vi "Set Password.vi"(11 "Ini File":path=path "D:/LABVIEW/SEQUENSER_SNA/Ver_12/INI/SysConfig.ini") -> (2 "Password":string, 3 "Password Ok":bool)   [LabVIEW 2018]
uses:
  <vilib>/Utility/miscctls.llb/LVSelectionTypeDef.ctl
  <vilib>/Utility/config.llb/Read Key (U32).vi
  <vilib>/Utility/config.llb/Read Key (String).vi
  <vilib>/Utility/config.llb/NI_LVConfig.lvlib
panel:
  out "Exit":bool
  out "Value":string
  out "Length":u32
  in  "stop":bool
  out "Key Focus":bool
  in  "Password In":string="****"
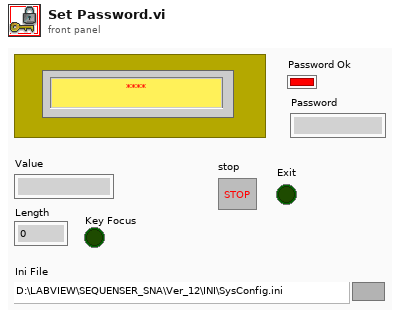
[diagram p1: front panel]
types:
  T1 = enum32{"Invalid", "Standard", "Closed", "Hidden", "Minimized", "Maximized"}
  T2 = enum32{"Invalid", "Default", "Floating", "Floating/Auto-Hide", "Modal"}
  T3 = typedef "LVSelectionTypeDef.ctl" = cluster{"Selection Start":u32, "Selection End":u32}
  T4 = typedef "NI_LVConfig.lvlib/Config Data RefNum.ctl" = refnum<k1>
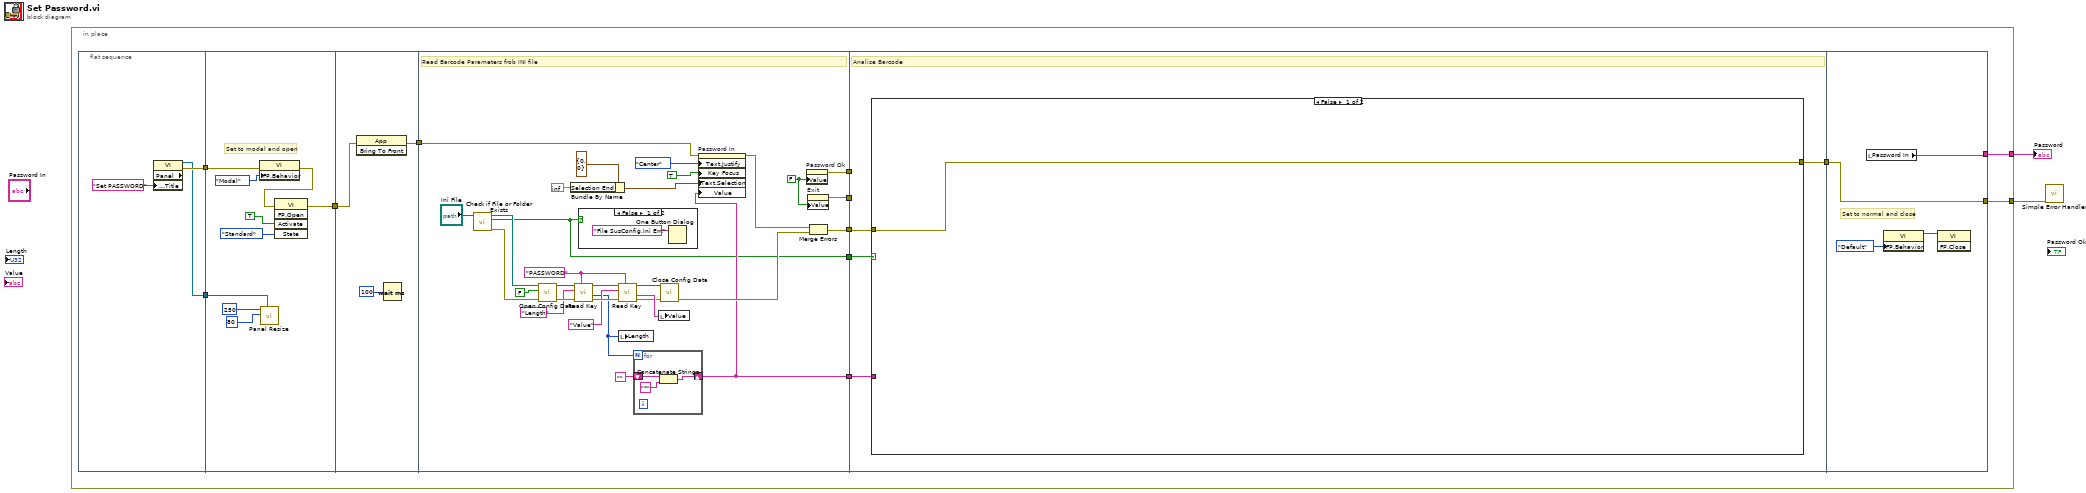
[diagram p0: block diagram]
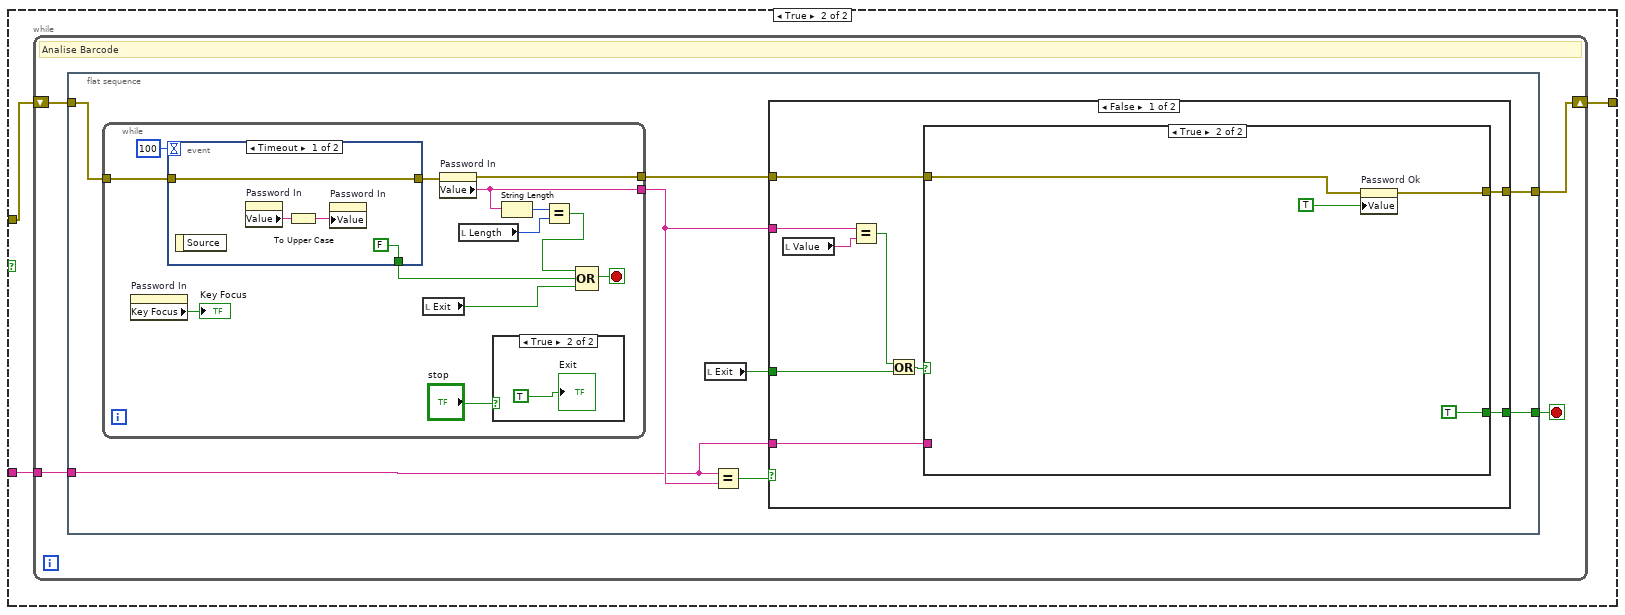
[diagram p3: hidden frame]
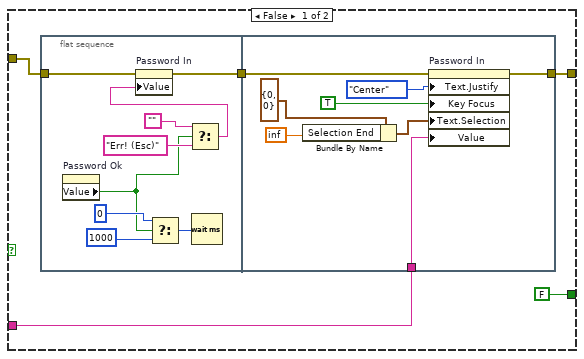
[diagram p4: hidden frame]
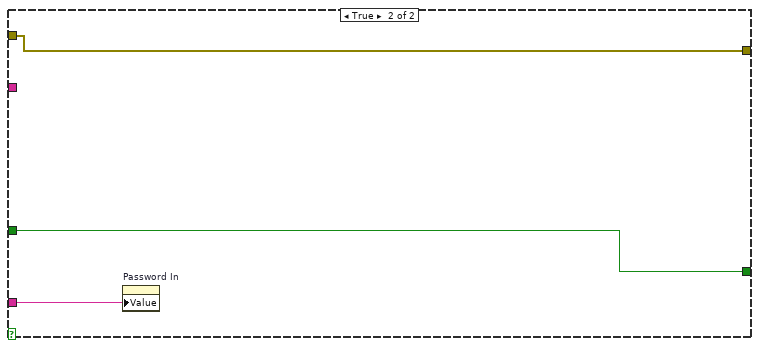
[diagram p5: hidden frame]
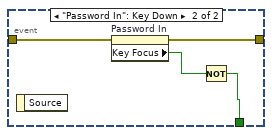
[diagram p7: hidden frame]
diagram:
  n1 = in-place {
    in-place-border: [w9] -> w2
    in-place-border: [w8] -> w1
    n2 = flat-sequence {
      tunnel: [w16] -> w14
      tunnel: [w15] -> w13
      tunnel: [w23] -> w12
      tunnel: w14 -> [w22]
      tunnel: w13 -> [w20]
      tunnel: [w29] -> w11
      tunnel: w12 -> [w27]
      tunnel: w11 -> [w45]
      tunnel: [w51] -> w10
      tunnel: [w44] -> w6
      tunnel: [w34] -> w5
      tunnel: [w32] -> w4
      tunnel: [w31] -> w3
      tunnel: w10 -> [w67]
      tunnel: [w66] -> w7
      tunnel: w6 -> [_]
      tunnel: w5 -> [w65]
      tunnel: w4 -> [_]
      tunnel: w3 -> [w64]
      tunnel: [w144] -> w9
      tunnel: [w146] -> w8
      tunnel: w7 -> [w144]
      frame #0 {
        n3 = property class="VI" props=["Panel", "Front Panel.Title"]("Front Panel.Title"="Set PASSWORD" ("Front Panel Window:Title")) -> (reference out=w15:refnum<vi>, error out=w16:errorcluster)  [unwired: 2 in, 1 out]
      }
      frame #1 {
        # "Set to modal and open"
        n4 = property class="VI"(error in=w22, "FP.Behavior"=T2."Modal" ("Front Panel Window:Behavior")) -> (error out=w26:errorcluster)  [unwired: 1 in, 1 out]
        n5 = call "Panel Resize.vi"("Width"=i16 250, "Height"=i16 80, "reference"=w20) -> ()  [unwired: 7 in, 1 out]
        n6 = invoke class="VI" method="FP.Open"(error in=w26, "Activate"=TRUE ("Activate?"), "State"=T1."Standard") -> (error out=w23:errorcluster)  [unwired: 2 in, 4 out]
      }
      frame #2 {
        n7 = invoke class="App" method="Bring To Front"(error in=w27) -> (error out=w29:errorcluster)  [unwired: 2 in, 2 out]
        n8 = Wait (ms)(milliseconds to wait=u32 100) -> ()  [unwired: 1 out]
      }
      frame #3 {
        w33 = FALSE ("Exit")
        w54 = "PASSWORD"
        # "Read Barcode Parameters frob INI file"
        n9 = call <vilib>:"Check if File or Folder Exists.vi"("path"="Ini File") -> ("error out"=w57:errorcluster, "file or folder exists?"=w31:bool, "dup path"=w58:path)  [unwired: 8 in]
        n10 = call <vilib>:"Open Config Data.vi"("error in (no error)"=w57, "create file if necessary (T)"=FALSE, "configuration file path"=w58) -> ("error out"=w52:errorcluster, "refnum"=w56:T4)  [unwired: 6 in, 1 out]
        n11 = Bundle By Name(cluster=T3 {"Selection Start"=0, "Selection End"=0} ("Text.Selection"), "Selection End"=inf) -> (w38:T3)
        n12 = call-poly <vilib>:"Read Key.vi"("section"=w54, "error in (no error)"=w52, "key"="Length", "refnum"=w56) -> ("error out"=w53:errorcluster, "value"=w36:u32, "refnum out"=w55:T4)  [unwired: 4 in, 1 out]
        n13 = case shown="False" w31 {
          frame False {
            n14 = One Button Dialog(message="File SusConfig.Ini Err!") -> ()  [unwired: 1 in, 1 out]
          }
          frame True {
          }
        }
        n15 = call-poly <vilib>:"Read Key.vi"("section"=w54, "error in (no error)"=w53, "key"="Value", "refnum"=w55) -> ("error out"=w42:errorcluster, "value"=w46:string, "refnum out"=w43:T4)  [unwired: 4 in, 1 out]
        n16 = local write "Length"(w36) -> ()
        n17 = for {
          N: w36 -> [_]
          shift-right: [w61] -> w34
          shift-left: "" -> [w62]
          n18 = Concatenate Strings(w62, "*") -> (w61:string)
        }
        n19 = local write "Value"(w46) -> ()
        n20 = call <vilib>:"Close Config Data.vi"("error in (no error)"=w42, "refnum"=w43) -> ("error out"=w49:errorcluster)  [unwired: 8 in, 1 out]
        n21 = property on="Password In" class="Str"(error in=w45, "Text.Justify"=enum16{"Left", "Center", "Right"}."Center" ("Text.Justification"), "Key Focus"=TRUE, "Text.Selection"=w38, "Value"=w34) -> (error out=w50:errorcluster)  [unwired: 1 in, 1 out]
        n22 = property on="Password Ok" class="Bool (strict)"("Value"=w33) -> (error out=w44:errorcluster)  [unwired: 2 in, 1 out]
        n23 = property on="Exit" class="Bool (strict)"("Value"=w33) -> (error out=w32:errorcluster)  [unwired: 2 in, 1 out]
        n24 = Merge Errors(w50, w49) -> (w51:errorcluster)
      }
      frame #4 {
        # "Analise Barcode"
        n25 = case shown="False" w64 {
          tunnel: w67 -> [w68 w71]
          tunnel: [w68 w70] -> w66
          tunnel: w65 -> [_ w69]
          frame False {
          }
          frame True {
            n26 = while {
              shift-right: [w73] -> w70
              shift-left: w71 -> [w75]
              tunnel: w69 -> [w72]
              stop <- w74 stop-if-true
              # "Analise Barcode"
              n27 = flat-sequence {
                tunnel: [w82] -> w74
                tunnel: [w81] -> w73
                tunnel: w75 -> [w83]
                tunnel: w72 -> [w77]
                frame #0 {
                  n28 = while {
                    tunnel: w83 -> [w132]
                    tunnel: [w129] -> w80
                    tunnel: [w128] -> w78
                    stop <- w123 stop-if-true
                    n29 = property on="Password In" class="Str"() -> ("Key Focus"=→"Key Focus":bool)  [unwired: 2 in, 2 out]
                    n30 = event shown="[0] Timeout" {
                      selector: _ -> [_ _]
                      dyn-events: _ -> [_ _]
                      timeout: 100 -> [_ _]
                      tunnel: [FALSE w142] -> w124
                      tunnel: w132 -> [w136 w141]
                      tunnel: [w136 w140] -> w130
                      event Timeout {
                        n31 = event-data() -> ()  [unwired: 1 in, 1 out]
                        n32 = property on="Password In" class="Str"() -> ("Value"=w139:string)  [unwired: 2 in, 2 out]
                        n33 = To Upper Case(1:w139) -> (0:w138:string)
                        n34 = property on="Password In" class="Str"("Value"=w138) -> ()  [unwired: 2 in, 2 out]
                      }
                      event "Password In": Key Down {
                        n35 = event-data() -> ()  [unwired: 1 in, 1 out]
                        n36 = property on="Password In" class="Str"(error in=w141) -> (error out=w140:errorcluster, "Key Focus"=w143:bool)  [unwired: 1 in, 1 out]
                        n37 = Not(x=w143) -> (.not. x?=w142:bool)
                      }
                    }
                    n38 = local read "Exit"() -> (w122:bool)
                    n39 = property on="Password In" class="Str"(error in=w130) -> (error out=w129:errorcluster, "Value"=w128:string)  [unwired: 1 in, 1 out]
                    n40 = local read "Length"() -> (w126:u32)
                    n41 = case shown="True" "stop" {
                      frame False {
                      }
                      frame True {
                        "Exit" <- TRUE ("Exit")
                      }
                    }
                    n42 = String Length(string=w128) -> (length=w127:i32)
                    n43 = Equal?(x=w127, y=w126) -> (x = y?=w125:bool)
                    n44 = Compound Arithmetic op=OR(w125, w124, w122) -> (w123:bool)
                  }
                  n45 = local read "Exit"() -> (w76:bool)
                  n46 = Equal?(x=w77, y=w78) -> (x = y?=w79:bool)
                  n47 = case shown="False" w79 {
                    tunnel: [w92 w119] -> w82
                    tunnel: [w91 w121] -> w81
                    tunnel: w80 -> [w89 w121]
                    tunnel: w78 -> [w88 _]
                    tunnel: w76 -> [w85 w119]
                    tunnel: w77 -> [w84 w120]
                    frame False {
                      n48 = local read "Value"() -> (w87:string)
                      n49 = Equal?(x=w88, y=w87) -> (x = y?=w86:bool)
                      n50 = Or(x=w86, y=w85) -> (x .or. y?=w90:bool)
                      n51 = case shown="True" w90 {
                        tunnel: [FALSE TRUE] -> w92
                        tunnel: [w96 w117] -> w91
                        tunnel: w89 -> [w94 w116]
                        tunnel: w84 -> [w93 _]
                        frame False {
                          n52 = flat-sequence {
                            tunnel: [w106] -> w95
                            tunnel: w94 -> [w105]
                            tunnel: [w112] -> w96
                            tunnel: w95 -> [w111]
                            tunnel: w93 -> [w107]
                            frame #0 {
                              n53 = property on="Password Ok" class="Bool (strict)"() -> ("Value"=w98:bool)  [unwired: 2 in, 2 out]
                              n54 = Select(t=u32 0 ("milliseconds to wait"), s=w98, f=u32 1000 ("milliseconds to wait")) -> (s? t:f=w101:u32)
                              n55 = Select(t="", s=w98, f="Err! (Esc)") -> (s? t:f=w104:string)
                              n56 = property on="Password In" class="Str"(error in=w105, "Value"=w104) -> (error out=w106:errorcluster)  [unwired: 1 in, 1 out]
                              n57 = Wait (ms)(milliseconds to wait=w101) -> ()  [unwired: 1 out]
                            }
                            frame #1 {
                              n58 = Bundle By Name(cluster=T3 {"Selection Start"=0, "Selection End"=0} ("Text.Selection"), "Selection End"=inf) -> (w109:T3)
                              n59 = property on="Password In" class="Str"(error in=w111, "Text.Justify"=enum16{"Left", "Center", "Right"}."Center" ("Text.Justification"), "Key Focus"=TRUE, "Text.Selection"=w109, "Value"=w107) -> (error out=w112:errorcluster)  [unwired: 1 in, 1 out]
                            }
                          }
                        }
                        frame True {
                          n60 = property on="Password Ok" class="Bool (strict)"(error in=w116, "Value"=TRUE ("Password Ok")) -> (error out=w117:errorcluster)  [unwired: 1 in, 1 out]
                        }
                      }
                    }
                    frame True {
                      n61 = property on="Password In" class="Str"("Value"=w120) -> ()  [unwired: 2 in, 2 out]
                    }
                  }
                }
              }
            }
          }
        }
      }
      frame #5 {
        # "Set to normal and close"
        n62 = local read "Password In"() -> (w146:string)
        n63 = property class="VI"("FP.Behavior"=T2."Default" ("Front Panel Window:Behavior")) -> (reference out=w145:refnum<vi>)  [unwired: 2 in, 1 out]
        n64 = invoke class="VI" method="FP.Close"(reference=w145) -> ()  [unwired: 2 in, 3 out]
      }
    }
  }
  "Password" <- w1
  n65 = call <vilib>:"Simple Error Handler.vi"("error in (no error)"=w2) -> ()  [unwired: 4 in, 5 out]
